vi "RegisterTrendPointsRoutedMessage_Name.vi"() -> (1 "message name":string)   [LabVIEW 2017, in "DataEventCreator.lvlib"]
uses:
  <vilib>/addons/InsightCM/Devices/Shared/Common/DataEventCreator/DataEventCreator.lvlib
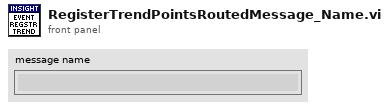
[diagram p1: front panel]
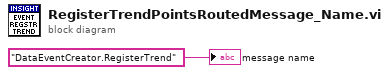
[diagram p0: block diagram]
diagram:
  "message name" <- "DataEventCreator.RegisterTrend" ("ProcessName")
